vi "FK 5-bar Mechanism.vi"(3 "error in (no error)":errorcluster, 4 "motors angles":dbl[](array[numeric])=[0.0, 0.0, 0.0, 0.0, 0.0, 0.0, 0.0], 5 "Finger in":refnum<class "Finger.lvclass">) -> (0 "error out":errorcluster, 1 "joint angles":dbl[](array[numeric]), 2 "Finger out":refnum<class "Finger.lvclass">)   [LabVIEW 2011, in "Finger.lvclass"]
uses:
  Finger.lvclass
  Finger.lvclass/Finger.ctl
panel:
  out "alpha":dbl
  out "theta":dbl
  out "psi":dbl
  out "phi":dbl
  out "d":dbl
  out "L4":dbl
  out "L3":dbl
  out "L2":dbl
  out "L1":dbl
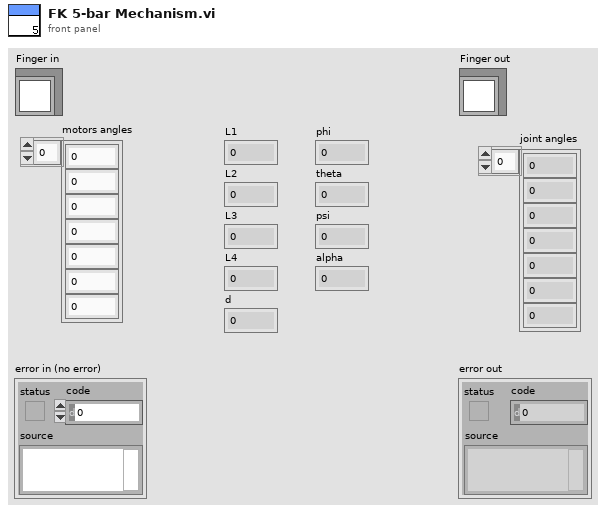
[diagram p1: front panel]
types:
  T1 = typedef "5-bar Side.ctl" = enum16{"Left", "Right"}
  T2 = cluster{"L1":dbl, "L2":dbl, "L3":dbl, "L4":dbl, "d":dbl}
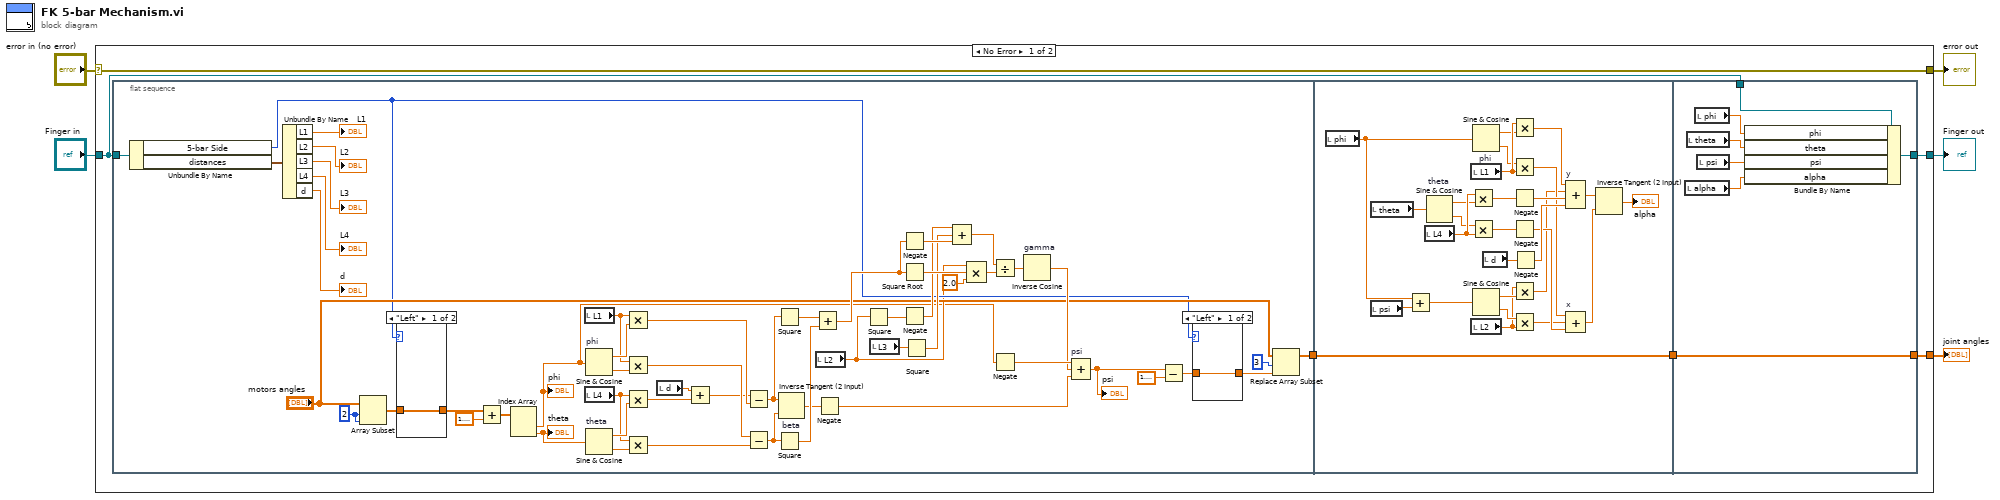
[diagram p0: block diagram]
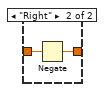
[diagram p2: hidden frame]
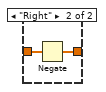
[diagram p3: hidden frame]
diagram:
  n1 = case shown="No Error" "error in (no error)" {
    selector: "error in (no error)" -> [w11 w107]
    tunnel: [w11 w107] -> w4
    tunnel: "Finger in" -> [w6 w106]
    tunnel: [w7 w106] -> w2
    tunnel: [w10 _] -> w1
    frame No Error {
      n2 = flat-sequence {
        tunnel: w6 -> [w27]
        tunnel: [w12] -> w9
        tunnel: w9 -> [w98]
        tunnel: [w98] -> w8
        tunnel: [w105] -> w10
        tunnel: w8 -> [w105]
        tunnel: [w100] -> w7
        tunnel: w6 -> [w99]
        frame #0 {
          w64 = 2 ("index")
          n3 = Unbundle By Name(w27) -> ("5-bar Side"=w26:T1, "distances"=w29:T2)
          n4 = Unbundle By Name(w29) -> ("L1"=→"L1":dbl, "L2"=→"L2":dbl, "L3"=→"L3":dbl, "L4"=→"L4":dbl, "d"=→"d":dbl)
          n5 = Array Subset(array="motors angles", index=w64, length=w64) -> (w31:dbl[])
          n6 = case shown="\"Left\"" w26 {
            tunnel: w31 -> [w69 w71]
            tunnel: [w69 w70] -> w30
            frame "Left" {
            }
            frame "Right" {
              n7 = Negate(x=w71) -> (-x=w70:dbl[])
            }
          }
          n8 = Add(x=w30, y=1.5707963267948966) -> (x+y=w32:dbl[])
          n9 = Index Array(array=w32) -> (element #1=w13:dbl, element #2=w14:dbl)  [unwired: 2 in]
          "phi" <- w13
          "theta" <- w14
          n10 = local read "L1"() -> (w23:dbl)
          n11 = local read "L4"() -> (w20:dbl)
          n12 = Sine & Cosine "phi"(0:w13) -> (1:w25:dbl, 2:w61:dbl)
          n13 = Sine & Cosine "theta"(0:w14) -> (1:w63:dbl, 2:w62:dbl)
          n14 = Multiply(x=w23, y=w25) -> (x*y=w38:dbl)
          n15 = Multiply(x=w23, y=w61) -> (x*y=w59:dbl)
          n16 = Multiply(x=w20, y=w63) -> (x*y=w37:dbl)
          n17 = Multiply(x=w20, y=w62) -> (x*y=w60:dbl)
          n18 = local read "d"() -> (w19:dbl)
          n19 = Add(x=w19, y=w37) -> (x+y=w36:dbl)
          n20 = Subtract(x=w36, y=w38) -> (x-y=w40:dbl)
          n21 = Subtract(x=w59, y=w60) -> (x-y=w39:dbl)
          n22 = Square(x=w40) -> (x^2=w58:dbl)
          n23 = Square(x=w39) -> (x^2=w57:dbl)
          n24 = Inverse Tangent (2 Input) "beta"(1:w39, 2:w40) -> (0:w46:dbl)
          n25 = Add(x=w58, y=w57) -> (x+y=w53:dbl)
          n26 = local read "L2"() -> (w24:dbl)
          n27 = Negate(x=w46) -> (-x=w43:dbl)
          n28 = Square(x=w24) -> (x^2=w55:dbl)
          n29 = local read "L3"() -> (w21:dbl)
          n30 = Negate(x=w53) -> (-x=w56:dbl)
          n31 = Square Root(x=w53) -> (sqrt(x)=w52:dbl)
          n32 = Negate(x=w55) -> (-x=w49:dbl)
          n33 = Square(x=w21) -> (x^2=w48:dbl)
          n34 = Compound Arithmetic op=ADD(w49, w48, w56) -> (w54:dbl)
          n35 = Compound Arithmetic op=MULTIPLY(w24, w52, 2.0 ("value")) -> (w50:dbl)
          n36 = Divide(x=w54, y=w50) -> (x/y=w47:dbl)
          n37 = Negate(x=w13) -> (-x=w45:dbl)
          n38 = Inverse Cosine "gamma"(1:w47) -> (0:w44:dbl)
          n39 = Compound Arithmetic op=ADD "psi"(w45, w44, w43) -> (w15:dbl)
          "psi" <- w15
          n40 = Subtract(x=w15, y=1.5707963267948966) -> (x-y=w33:dbl)
          n41 = case shown="\"Left\"" w26 {
            tunnel: w33 -> [w66 w68]
            tunnel: [w66 w67] -> w35
            frame "Left" {
            }
            frame "Right" {
              n42 = Negate(x=w68) -> (-x=w67:dbl)
            }
          }
          n43 = Replace Array Subset(array="motors angles", new element=w35, index=3) -> (w12:dbl[])
        }
        frame #1 {
          n44 = local read "phi"() -> (w78:dbl)
          n45 = local read "theta"() -> (w84:dbl)
          n46 = local read "psi"() -> (w79:dbl)
          n47 = Add(x=w78, y=w79) -> (x+y=w77:dbl)
          n48 = local read "L4"() -> (w90:dbl)
          n49 = Sine & Cosine "theta"(0:w84) -> (1:w88:dbl, 2:w89:dbl)
          n50 = Multiply(x=w90, y=w88) -> (x*y=w91:dbl)
          n51 = Multiply(x=w89, y=w90) -> (x*y=w94:dbl)
          n52 = local read "L1"() -> (w87:dbl)
          n53 = local read "L2"() -> (w74:dbl)
          n54 = Sine & Cosine "phi"(0:w78) -> (1:w85:dbl, 2:w86:dbl)
          n55 = Sine & Cosine(0:w77) -> (1:w75:dbl, 2:w76:dbl)
          n56 = local read "d"() -> (w97:dbl)
          n57 = Multiply(x=w87, y=w85) -> (x*y=w93:dbl)
          n58 = Multiply(x=w86, y=w87) -> (x*y=w80:dbl)
          n59 = Negate(x=w91) -> (-x=w92:dbl)
          n60 = Negate(x=w94) -> (-x=w95:dbl)
          n61 = Multiply(x=w74, y=w75) -> (x*y=w73:dbl)
          n62 = Multiply(x=w76, y=w74) -> (x*y=w72:dbl)
          n63 = Negate(x=w97) -> (-x=w96:dbl)
          n64 = Compound Arithmetic op=ADD "y"(w93, w73, w92, w96) -> (w81:dbl)
          n65 = Compound Arithmetic op=ADD "x"(w80, w72, w95) -> (w82:dbl)
          n66 = Inverse Tangent (2 Input)(1:w82, 2:w81) -> (0:→"alpha":dbl)
        }
        frame #2 {
          n67 = local read "alpha"() -> (w104:dbl)
          n68 = local read "theta"() -> (w102:dbl)
          n69 = local read "phi"() -> (w101:dbl)
          n70 = local read "psi"() -> (w103:dbl)
          n71 = Bundle By Name(cluster=w99, "phi"=w101, "theta"=w102, "psi"=w103, "alpha"=w104) -> (w100:refnum<class "Finger.lvclass">)
        }
      }
    }
    frame Error {
    }
  }
  "error out" <- w4
  "Finger out" <- w2
  "joint angles" <- w1
